vi "Validate Series CFG.vi"(8 "error in":errorcluster, 11 "<JSON>":string) -> (0 "error out":errorcluster, 2 "Is Valid?":bool)   [LabVIEW 2023, in "Configuration UI Actor.lvlib" / "Configuration UI Actor.lvclass"]
uses:
  Configuration UI Actor.lvclass
  MAL/Series/Series Actor/Series Actor/Series Actor.lvclass
  MAL/Task/Task Actor/Task Actor/Task Actor.lvclass
  525388c0-5307-449e-a095-feab6bb15fee.vi
  cd495714-564a-4e44-a0e5-1f4e0ab9e53b.vi
  525388c0-5307-449e-a095-feab6bb15fee.vi/a4169a97-72fc-4003-a778-603cf20cafa0.vi
  cd495714-564a-4e44-a0e5-1f4e0ab9e53b.vi/a4169a97-72fc-4003-a778-603cf20cafa0.vi
  <vilib>/JDP Science/JSONtext/Find Item.vi
  <vilib>/JDP Science/JSONtext/Next JSON Value.vi
  <vilib>/JDP Science/JSONtext/String Subset.vi
  <vilib>/JDP Science/JSONtext/Parsing/Advance past next JSON Value (inlined COPY).vi
  <vilib>/JDP Science/JSONtext/Parsing/Advance past whitespace.vi
  <vilib>/JDP Science/JSONtext/Parsing/Advance past String.vi
  <vilib>/JDP Science/JSONtext/Parsing/Advance past Number.vi
  <vilib>/JDP Science/JSONtext/Parsing/Advance past Line Ending.vi
  <vilib>/JDP Science/JSONtext/Parsing/Parse Full Path or Item Name.vi
  <vilib>/JDP Science/JSONtext/Parsing/Advance past Array.vi
  <vilib>/JDP Science/JSONtext/Parsing/Advance past Object.vi
  <vilib>/JDP Science/JSONtext/support/Error Cluster From Code.vi
  <vilib>/JDP Science/JSONtext/Offset/Find Item Locations by Path.vi
  <vilib>/JDP Science/JSONtext/JSON text to Variant.vi
  <vilib>/Utility/error.llb/Error Cluster From Error Code.vi
  <vilib>/JDP Science/JSONtext/LVClass Serializer/JSONtext LVClass Serializer.lvclass
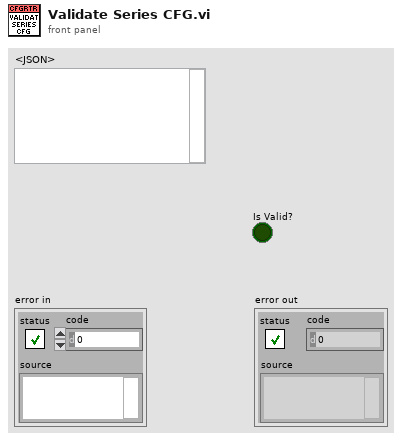
[diagram p1: front panel]
types:
  T1 = cluster{"Ident":string, "Class":string, "Point Idents":string[]}[]
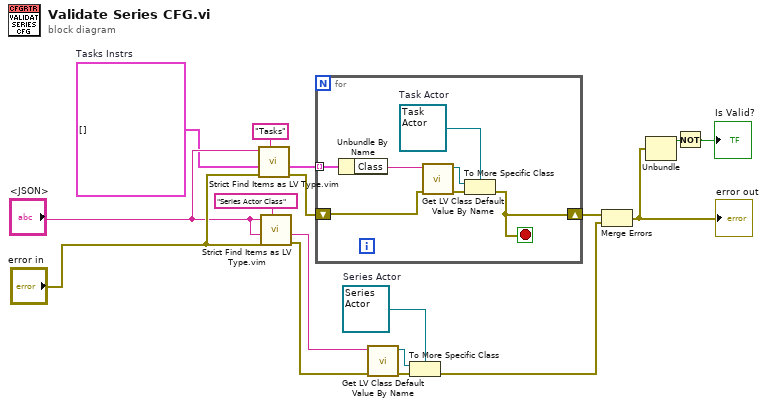
[diagram p0: block diagram]
diagram:
  w7 = T1 []  # Tasks Instrs
  w9 = refnum<class "Series Actor.lvclass"> refnum  # Series Actor
  n1 = call "Strict Find Items as LV Type.vim"("$Path or Item Name"="Tasks", "error in"="error in", "Data Type and Default Value"=w7, "<JSON>"="<JSON>") -> ("error out"=w17:errorcluster, "Data out"=w16:T1)  [unwired: 5 in, 1 out]
  n2 = call "Strict Find Items as LV Type.vim"("$Path or Item Name"="Series Actor Class", "error in"="error in", "Data Type and Default Value"="<JSON>", "<JSON>"="<JSON>") -> ("error out"=w13:errorcluster, "Data out"=w10:string)  [unwired: 5 in, 1 out]
  n3 = for {
    tunnel: w16 -> [w22] mode=indexing
    shift-right: [w18] -> w8
    shift-left: w17 -> [w20]
    stop <- w18 stop-if-true
    w19 = refnum<class "Task Actor.lvclass"> refnum  # Task Actor
    n4 = Unbundle By Name(w22) -> ("Class"=w21:string)
    n5 = call <vilib>:"Get LV Class Default Value By Name.vi"("error in (no error)"=w20, "class name"=w21) -> ("error out"=w24:errorcluster, "object"=w23:refnum<class>)  [unwired: 8 in]
    n6 = To More Specific Class(target class=w19, reference=w23, error in=w24) -> (error out=w18:errorcluster)  [unwired: 1 out]
  }
  n7 = call <vilib>:"Get LV Class Default Value By Name.vi"("error in (no error)"=w13, "class name"=w10) -> ("error out"=w11:errorcluster, "object"=w12:refnum<class>)  [unwired: 8 in]
  n8 = To More Specific Class(target class=w9, reference=w12, error in=w11) -> (error out=w4:errorcluster)  [unwired: 1 out]
  n9 = Merge Errors(w8, w4) -> (w3:errorcluster)
  "error out" <- w3
  n10 = Unbundle(w3) -> ("status"=w2:bool)  [unwired: 2 out]
  n11 = Not(x=w2) -> (.not. x?=→"Is Valid?":bool)
